vi "AB_Source_Set_Property.vi"(8 "error in (no error)":errorcluster, 10 "sourceProperty":T1={"sourcePropertyType"=enum."Password", "value"=variant}, 11 "sourceProperties in":T1[](array[typedef])) -> (0 "error out":errorcluster, 2 "replaced":bool, 3 "sourceProperties out":T1[](array[typedef]))   [LabVIEW 2020]
uses:
  <vilib>/AppBuilder/AB_Source_Properties.ctl
  <vilib>/AppBuilder/AB_Source_Property_Type.ctl
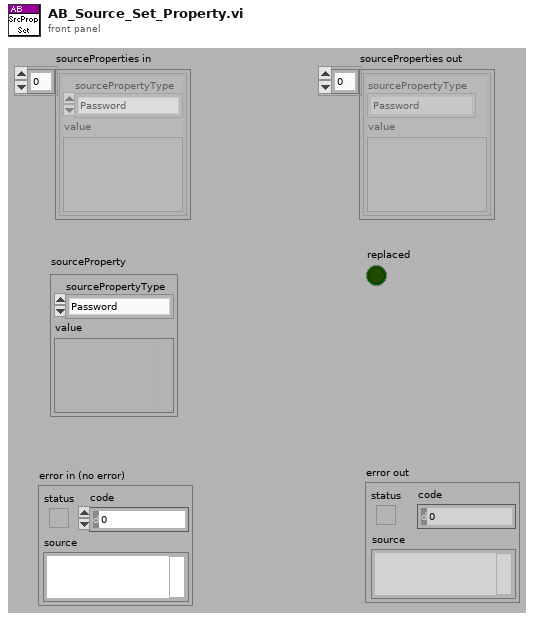
[diagram p1: front panel]
types:
  T1 = typedef "AB_Source_Properties.ctl" = cluster{"sourcePropertyType":T2, "value":variant}
  T2 = typedef "AB_Source_Property_Type.ctl" = enum16{"Remove block diagram", "Remove front panel", "Password", "Window has title bar", "Show menu bar", "Show vertical scroll bar", "Show horizontal scroll bar", "Show toolbar", "Show Abort button", "Show fp when called", "Window behavior", "Allow user to close window", "Window run-time position", "Run when opened", "Allow debugging", "Auto error handling", "Generate guard code", "Use stack variables", "Expression folding", "Integer only", "Inline subVI"}
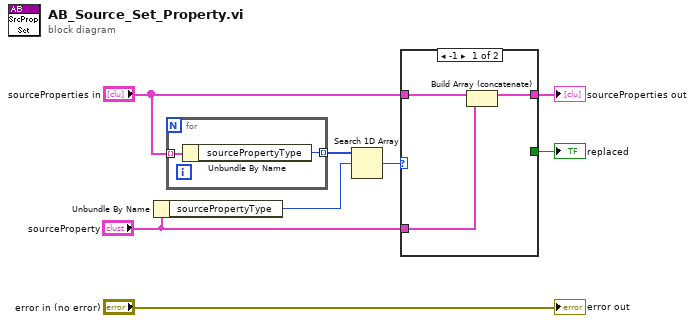
[diagram p0: block diagram]
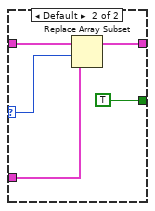
[diagram p2: hidden frame]
diagram:
  n1 = Unbundle By Name("sourceProperty") -> ("sourcePropertyType"=w3:T2)
  n2 = for {
    tunnel: "sourceProperties in" -> [w10] mode=indexing
    tunnel: [w9] -> w8 mode=indexing
    n3 = Unbundle By Name(w10) -> ("sourcePropertyType"=w9:T2)
  }
  n4 = Search 1D Array(1D array=w8, element=w3) -> (index of element=w7:i32)  [unwired: 1 in]
  n5 = case shown="-1" w7 {
    selector: w7 -> [_ w15]
    tunnel: "sourceProperties in" -> [w13 w17]
    tunnel: [_ TRUE] -> w5
    tunnel: [w11 w16] -> w2
    tunnel: "sourceProperty" -> [w12 w14]
    frame -1 {
      n6 = Build Array (concatenate)(w13, w12) -> (w11:T1[])
    }
    frame Default {
      n7 = Replace Array Subset(array=w17, new element=w14, index=w15) -> (w16:T1[])
    }
  }
  "sourceProperties out" <- w2
  "replaced" <- w5
  "error out" <- "error in (no error)"
